vi "isRootDir.vi"(11 "path":path=path "\\\\cn-xia-fs1\\Incoming/yaoli") -> (3 "Boolean":bool)   [LabVIEW 2017, in "application.lvlib" / "application.lvclass"]
uses:
  application.lvclass
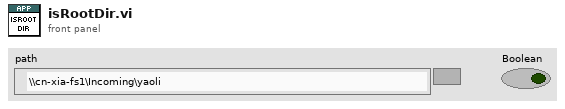
[diagram p1: front panel]
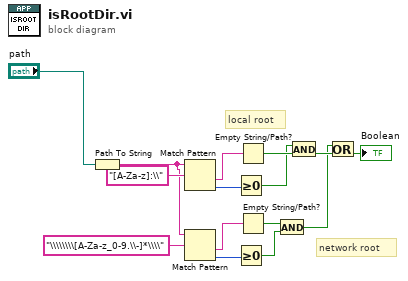
[diagram p0: block diagram]
diagram:
  # "local root"
  # "network root"
  n1 = Path To String(path="path") -> (string=w6:string)
  n2 = Match Pattern(string=w6, regular expression="[A-Za-z]:\\") -> (after substring=w13:string, offset past match=w15:i32)  [unwired: 1 in, 2 out]
  n3 = Match Pattern(string=w6, regular expression="\\\\\\\\[A-Za-z_0-9.\\-]*\\\\") -> (after substring=w9:string, offset past match=w7:i32)  [unwired: 1 in, 2 out]
  n4 = Greater Or Equal To 0?(x=w15) -> (x >= 0?=w10:bool)
  n5 = Greater Or Equal To 0?(x=w7) -> (x >= 0?=w4:bool)
  n6 = Empty String/Path?(string/path=w13) -> (empty?=w12:bool)
  n7 = Empty String/Path?(string/path=w9) -> (empty?=w5:bool)
  n8 = And(x=w5, y=w4) -> (x .and. y?=w2:bool)
  n9 = And(x=w10, y=w12) -> (x .and. y?=w11:bool)
  n10 = Or(x=w2, y=w11) -> (x .or. y?=→"Boolean":bool)
